vi "Set From.vi"(8 "error in (no error)":errorcluster, 10 "From":T1, 11 "Gmail in":refnum<class "Gmail.lvclass">) -> (0 "error out":errorcluster, 3 "Gmail out":refnum<class "Gmail.lvclass">)   [LabVIEW 2020, in "Gmail API.lvlib" / "Gmail.lvclass"]
doc: "Sets the From address of the email. This is useful for setting the displayed name alongside the email. The email address must match the account authorized to send emails."
uses:
  Gmail.lvclass
  Mail Address.ctl
  Gmail.lvclass/Gmail.ctl
  Gmail API.lvlib
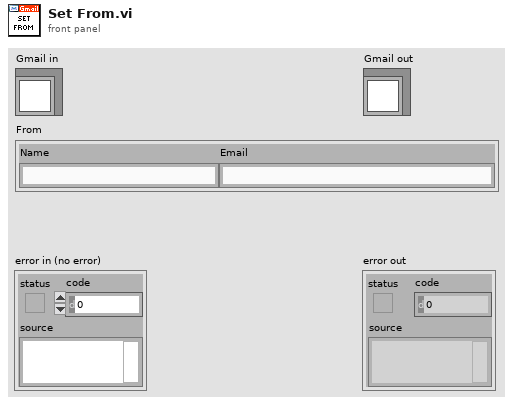
[diagram p1: front panel]
types:
  T1 = typedef "Gmail API.lvlib/Mail Address.ctl" = cluster{"Name":string, "Email":string}
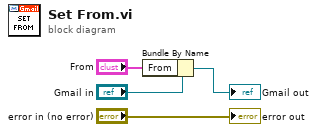
[diagram p0: block diagram]
diagram:
  n1 = Bundle By Name(cluster="Gmail in", "From"="From") -> (→"Gmail out":refnum<class "Gmail.lvclass">)
  "error out" <- "error in (no error)"
